vi "Set Stop Event.vi"(8 "error in (no error)":errorcluster, 10 "Server Stop Event":refnum<user-event>, 11 "Base Server in":refnum<class "Server.lvclass">) -> (0 "error out":errorcluster, 3 "Base Server out":refnum<class "Server.lvclass">)   [LabVIEW 2024, in "Ramses Framework.lvlib" / "Server.lvclass"]
uses:
  Server.lvclass
  Server.lvclass/Server.ctl
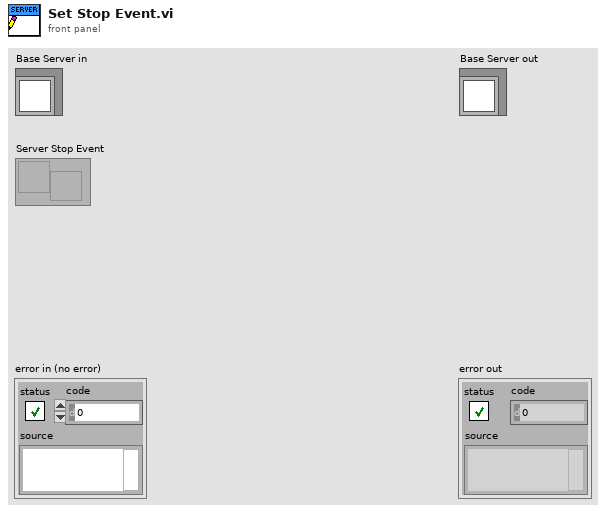
[diagram p1: front panel]
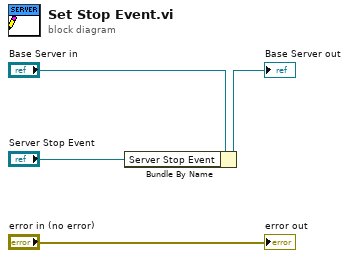
[diagram p0: block diagram]
diagram:
  n1 = Bundle By Name(cluster="Base Server in", "Server Stop Event"="Server Stop Event") -> (→"Base Server out":refnum<class "Server.lvclass">)
  "error out" <- "error in (no error)"
